vi "RestoreSetupLVSource.vi"(10 "Manual Test":bool) -> (0 "error out":errorcluster)   [LabVIEW 2020]
uses:
  <vilib>/Wiresmith Technology/G CLI/CLI Class/CLI.lvclass
  <vilib>/zip/NI_Unzip.lvlib
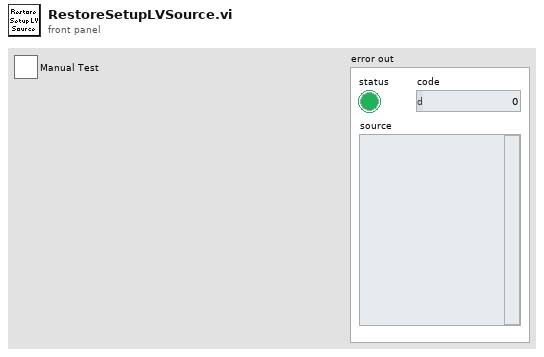
[diagram p1: front panel]
types:
  T1 = enum32{"Invalid", "Standard", "Closed", "Hidden", "Minimized", "Maximized"}
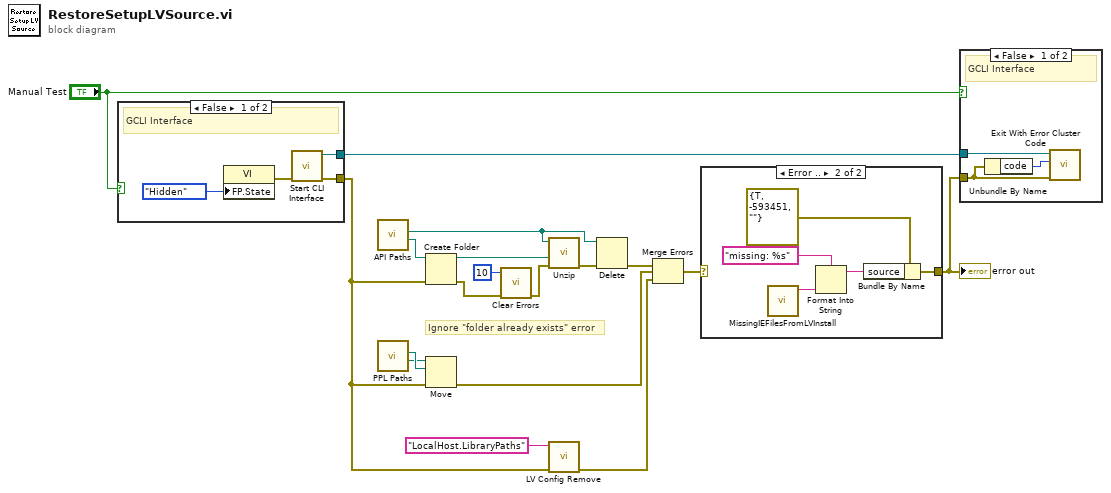
[diagram p0: block diagram]
diagram:
  # "Ignore \"folder already exists\" error"
  n1 = case shown="False" "Manual Test" {
    tunnel: [w21 _] -> w15
    tunnel: [w19 _] -> w1
    frame False {
      # "GCLI Interface"
      n2 = property class="VI"("FP.State"=T1."Hidden" ("Front Panel Window:State")) -> (error out=w22:errorcluster)  [unwired: 2 in, 1 out]
      n3 = call <vilib>:"Start CLI Interface.vi"("error in (no error)"=w22) -> ("error out"=w21:errorcluster, "CLI out"=w19:refnum<class "CLI.lvclass">)  [unwired: 7 in, 2 out]
    }
    frame True {
      # "Running Manual"
    }
  }
  n4 = call "API Paths.vi"() -> ("API Folder"=w7:path, "API Zip File"=w8:path)  [unwired: 10 in]
  n5 = call "PPL Paths.vi"() -> ("Renamed PPL Path"=w4:path, "PPL Path"=w5:path)  [unwired: 10 in]
  n6 = Create Folder(path (use dialog)=w7, error in=w15) -> (created path=w9:path, error out=w18:errorcluster)  [unwired: 1 in, 1 out]
  n7 = Move(source path=w4, error in=w15, 10:w5) -> (error out=w13:errorcluster)  [unwired: 2 in, 2 out]
  n8 = call <vilib>:"Clear Errors.vi"("error in (no error)"=w18, "specific error code to clear (0: all)"=10) -> ("error out"=w17:errorcluster)  [unwired: 4 in, 1 out]
  n9 = call <vilib>:"Unzip.vi"("error in (no error)"=w17, "Target directory (same as Zip file if empty)"=w9, "Zip file"=w8) -> ("error out"=w16:errorcluster)  [unwired: 6 in, 2 out]
  n10 = call <resource>:"LV Config Remove.vi"("error in"=w15, "key"="LocalHost.LibraryPaths") -> ("error out"=w12:errorcluster)  [unwired: 5 in]
  n11 = Delete(path (use dialog)=w8, error in=w16) -> (error out=w14:errorcluster)  [unwired: 3 in, 2 out]
  n12 = Merge Errors(w14, w13, w12) -> (w11:errorcluster)
  n13 = case shown="Error .." w11 {
    selector: w11 -> [w23 _]
    tunnel: [w23 w27] -> w10
    frame No Error {
    }
    frame Error {
      n14 = call "MissingIEFilesFromLVInstall.vi"() -> ("Missing IE Paths"=w24:string)  [unwired: 10 in, 1 out]
      n15 = Format Into String(format string="missing: %s" ("source"), w24) -> (resulting string=w25:string)  [unwired: 2 in, 1 out]
      n16 = Bundle By Name(cluster=errorcluster {"status"=TRUE, "code"=-593451, "source"=""} ("error out"), "source"=w25) -> (w27:errorcluster)
    }
  }
  "error out" <- w10
  n17 = case shown="False" "Manual Test" {
    tunnel: w1 -> [w30 _]
    tunnel: w10 -> [w31 _]
    frame False {
      # "GCLI Interface"
      n18 = Unbundle By Name(w31) -> ("code"=w29:i32)
      n19 = call <vilib>:"Exit With Error Cluster Code.vi"("error in (no error)"=w31, "No Error Code (0)"=w29, "CLI in"=w30) -> ()  [unwired: 8 in, 1 out]
    }
    frame True {
      # "Running Manual"
    }
  }
